vi "convert.messages.to.byteArray.vi"(11 "Messages.In":refnum<class "SequencedUnitHeader.lvclass">[](array[class])) -> (2 "ByteArray.out":u8[](array[numeric]) format="%.0x", 3 "2D.ByteArray.out":u8[][](array[numeric]))   [LabVIEW 2022 SP3]
uses:
  pitch/SequencedUnitHeader/SequencedUnitHeader.lvclass
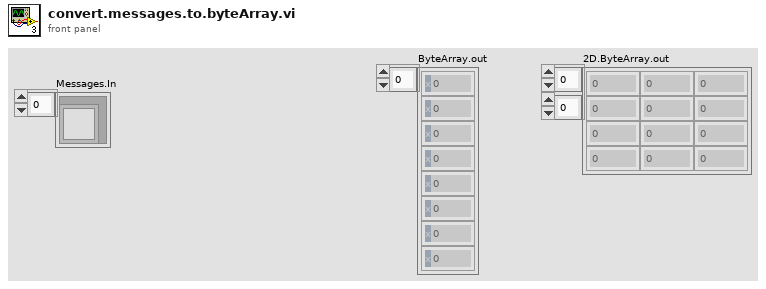
[diagram p1: front panel]
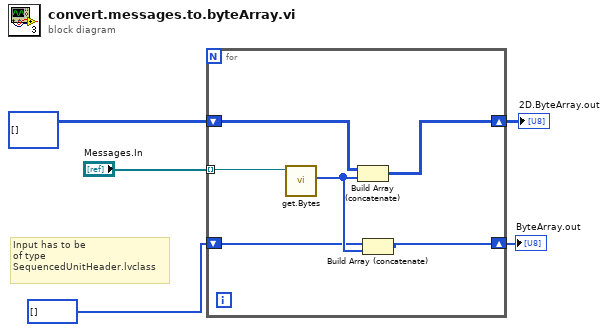
[diagram p0: block diagram]
diagram:
  # "Input has to be\nof type\nSequencedUnitHeader.lvclass"
  n1 = for {
    tunnel: "Messages.In" -> [w11] mode=indexing
    shift-right: [w9] -> w3
    shift-left: u8[][] [] -> [w10]
    shift-right: [w7] -> w1
    shift-left: u8[] [] -> [w6]
    n2 = call-dynamic "get.Bytes.vi"("SequencedUnitHeader in"=w11) -> ("Bytes.Out"=w8:u8[])  [unwired: 8 in, 2 out]
    n3 = Build Array (concatenate)(w10, w8) -> (w9:u8[][])
    n4 = Build Array (concatenate)(w6, w8) -> (w7:u8[])
  }
  "2D.ByteArray.out" <- w3
  "ByteArray.out" <- w1
